vi "tb_ 2 bit counter.vi"() -> ()   [LabVIEW 2011]
panel:
  out "Data":fxp<+,6,6>[](array[numeric])
  out "TC":bool[](array[boolean])
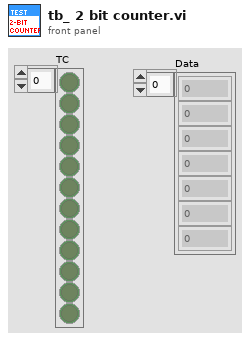
[diagram p1: front panel]
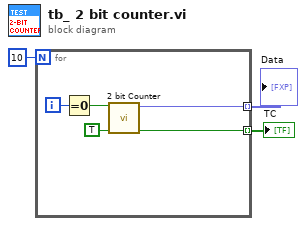
[diagram p0: block diagram]
diagram:
  n1 = for {
    N: 10 -> [_]
    tunnel: [w7] -> w1 mode=indexing
    tunnel: [w6] -> w3 mode=indexing
    i -> [w5]
    n2 = Equal To 0?(x=w5) -> (x = 0?=w4:bool)
    n3 = call "2 bit Counter.vi"("Increment?"=TRUE, "Reset?"=w4) -> ("terminal count"=w6:bool, "counter value"=w7:fxp<+,2,2>)  [unwired: 8 in]
  }
  "TC" <- w3
  "Data" <- w1
